vi "SaveOverlap.vi"(0 "ROI Cluster":T1, 1 "Intensity":dbl[][](array[numeric]), 2 "Auto Scale?":bool, 3 "Threshold (max)":dbl, 4 "Threshold (min)":dbl, 5 "G Data":dbl[][](array[numeric]), 6 "S Data":dbl[][](array[numeric]), 7 "error in":errorcluster, 8 "File Name":string, 9 "Index Name":string, 10 "Experiment Name":string, 11 "Time Stamp?":bool, 12 "Identify Name":string, 13 "Enable?":bool, 14 "path":path, 15 "Crop Pixels":u16=40) -> (20 "cancelled":bool, 27 "error out":errorcluster)   [LabVIEW 2018]
uses:
  <vilib>/picture/picture.llb/Draw True-Color Pixmap.vi
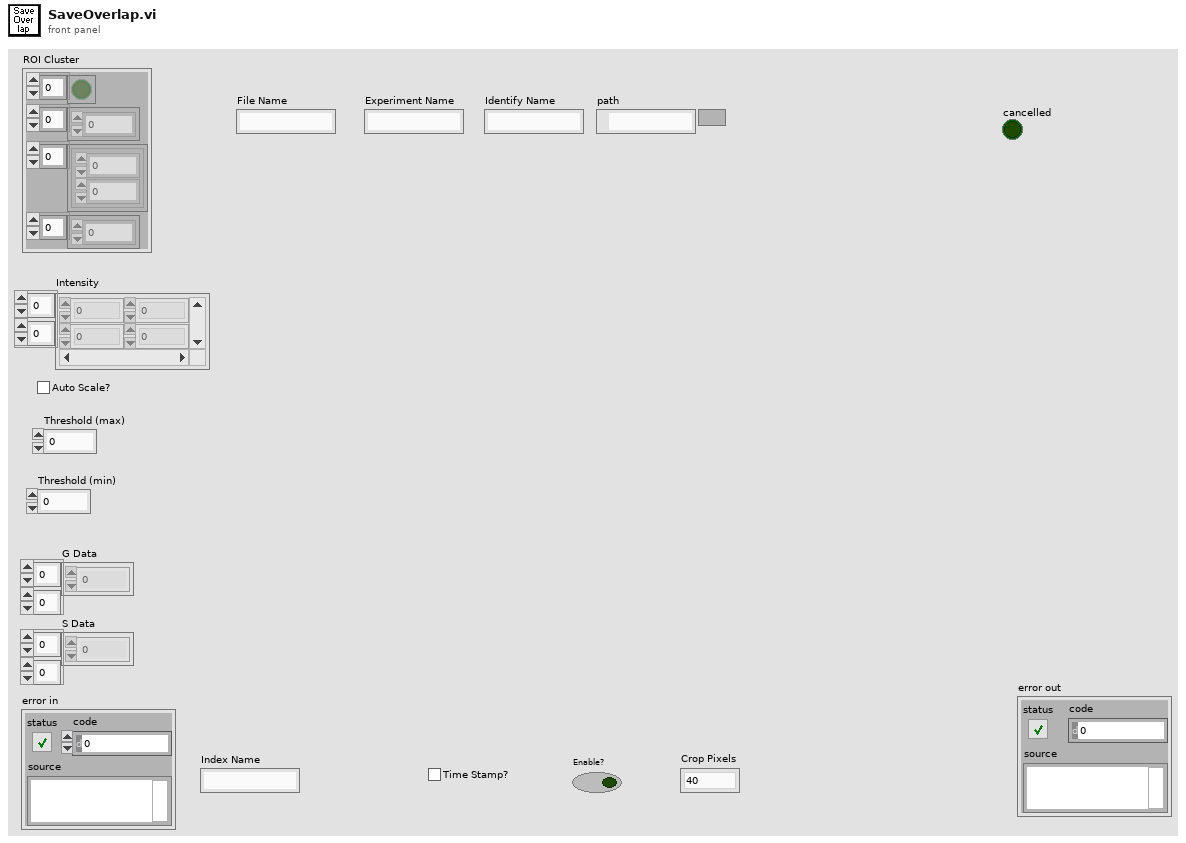
[diagram p1: front panel]
types:
  T1 = cluster{bool[], dbl[], cluster{dbl, dbl}[], u32[]}
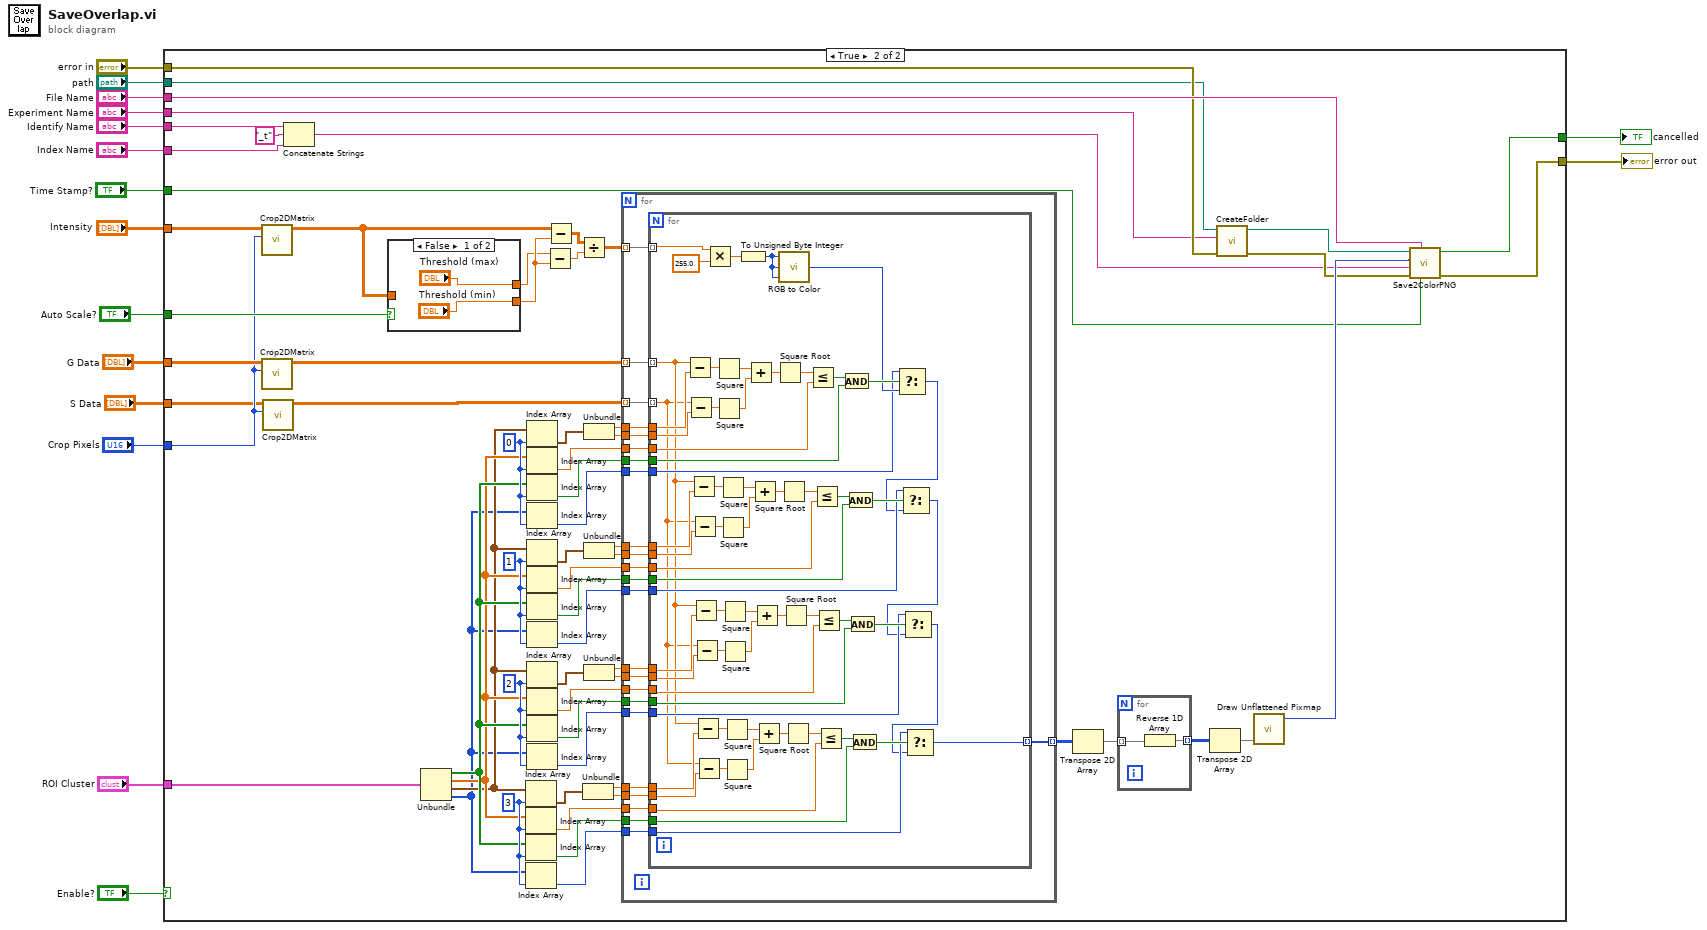
[diagram p0: block diagram]
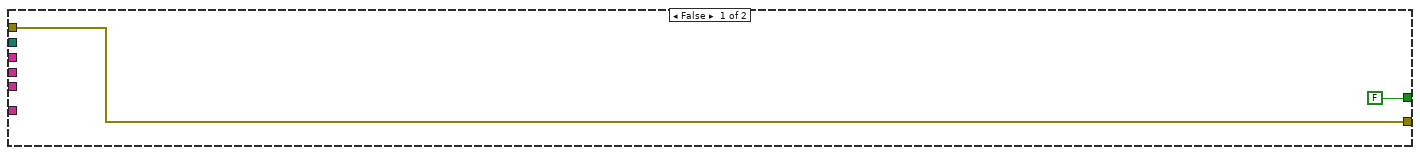
[diagram p2: hidden frame]
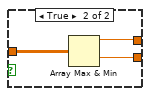
[diagram p3: hidden frame]
diagram:
  n1 = case shown="True" "Enable?" {
    tunnel: "S Data" -> [_ w30]
    tunnel: "G Data" -> [_ w33]
    tunnel: "Auto Scale?" -> [_ w78]
    tunnel: "Intensity" -> [_ w35]
    tunnel: "ROI Cluster" -> [_ w44]
    tunnel: "error in" -> [w17 w28]
    tunnel: [FALSE ("save cancelled") w38] -> w10
    tunnel: [w17 w39] -> w9
    tunnel: "path" -> [_ w27]
    tunnel: "File Name" -> [_ w37]
    tunnel: "Experiment Name" -> [_ w26]
    tunnel: "Identify Name" -> [_ w21]
    tunnel: "Time Stamp?" -> [_ w25]
    tunnel: "Crop Pixels" -> [_ w31]
    tunnel: "Index Name" -> [_ w20]
    frame False {
    }
    frame True {
      w47 = 3 ("index")
      w56 = 2 ("index")
      w61 = 1 ("index")
      w70 = 0 ("index")
      n2 = call "Crop2DMatrix.vi"("Crop Pixels"=w31, "Data"=w35) -> ("Cropped Data"=w34:dbl[][])  [unwired: 9 in]
      n3 = call "Crop2DMatrix.vi"("Crop Pixels"=w31, "Data"=w33) -> ("Cropped Data"=w32:dbl[][])  [unwired: 9 in]
      n4 = call "Crop2DMatrix.vi"("Crop Pixels"=w31, "Data"=w30) -> ("Cropped Data"=w29:dbl[][])  [unwired: 9 in]
      n5 = Concatenate Strings(w21, "_t" ("string"), w20) -> (w19:string)
      n6 = case shown="False" w78 {
        tunnel: w34 -> [_ w89]
        tunnel: ["Threshold (max)" w88] -> w76
        tunnel: ["Threshold (min)" w87] -> w77
        frame False {
        }
        frame True {
          n7 = Array Max & Min(array=w89) -> (max value=w88:dbl, min value=w87:dbl)  [unwired: 2 out]
        }
      }
      n8 = Unbundle(w44) -> (w43:bool[], w42:dbl[], w41:cluster{dbl, dbl}[], w40:u32[])
      n9 = Index Array(array=w41, index=w47) -> (element=w48:cluster{dbl, dbl})
      n10 = Index Array(array=w42, index=w47) -> (element=w49:dbl)
      n11 = Index Array(array=w43, index=w47) -> (element=w50:bool)
      n12 = Index Array(array=w40, index=w47) -> (element=w51:u32)
      n13 = Index Array(array=w41, index=w70) -> (element=w69:cluster{dbl, dbl})
      n14 = Index Array(array=w42, index=w70) -> (element=w68:dbl)
      n15 = Index Array(array=w43, index=w70) -> (element=w67:bool)
      n16 = Index Array(array=w40, index=w70) -> (element=w66:u32)
      n17 = Index Array(array=w41, index=w61) -> (element=w62:cluster{dbl, dbl})
      n18 = Index Array(array=w42, index=w61) -> (element=w63:dbl)
      n19 = Index Array(array=w43, index=w61) -> (element=w64:bool)
      n20 = Index Array(array=w40, index=w61) -> (element=w65:u32)
      n21 = Index Array(array=w41, index=w56) -> (element=w55:cluster{dbl, dbl})
      n22 = Index Array(array=w42, index=w56) -> (element=w54:dbl)
      n23 = Index Array(array=w43, index=w56) -> (element=w53:bool)
      n24 = Index Array(array=w40, index=w56) -> (element=w52:u32)
      n25 = Subtract(x=w76, y=w77) -> (x-y=w80:dbl)
      n26 = Subtract(x=w34, y=w77) -> (x-y=w79:dbl[][])
      n27 = Divide(x=w79, y=w80) -> (x/y=w72:dbl[][])
      n28 = Unbundle(w48) -> (w45:dbl, w46:dbl)
      n29 = Unbundle(w69) -> (w82:dbl, w81:dbl)
      n30 = Unbundle(w62) -> (w59:dbl, w60:dbl)
      n31 = Unbundle(w55) -> (w58:dbl, w57:dbl)
      n32 = for {
        tunnel: w32 -> [w113] mode=indexing
        tunnel: w29 -> [w112] mode=indexing
        tunnel: w82 -> [w111]
        tunnel: w81 -> [w110]
        tunnel: w68 -> [w109]
        tunnel: w72 -> [w108] mode=indexing
        tunnel: [w107] -> w71 mode=indexing
        tunnel: w67 -> [w106]
        tunnel: w66 -> [w105]
        tunnel: w59 -> [w100]
        tunnel: w60 -> [w101]
        tunnel: w63 -> [w102]
        tunnel: w64 -> [w103]
        tunnel: w65 -> [w104]
        tunnel: w58 -> [w99]
        tunnel: w57 -> [w98]
        tunnel: w54 -> [w97]
        tunnel: w53 -> [w96]
        tunnel: w52 -> [w95]
        tunnel: w45 -> [w90]
        tunnel: w46 -> [w91]
        tunnel: w49 -> [w92]
        tunnel: w50 -> [w93]
        tunnel: w51 -> [w94]
        n33 = for {
          tunnel: w113 -> [w119] mode=indexing
          tunnel: w112 -> [w118] mode=indexing
          tunnel: w111 -> [w176]
          tunnel: w110 -> [w175]
          tunnel: w109 -> [w174]
          tunnel: w108 -> [w164] mode=indexing
          tunnel: [w114] -> w107 mode=indexing
          tunnel: w106 -> [w162]
          tunnel: w105 -> [w159]
          tunnel: w100 -> [w150]
          tunnel: w101 -> [w149]
          tunnel: w102 -> [w148]
          tunnel: w103 -> [w147]
          tunnel: w104 -> [w146]
          tunnel: w99 -> [w129]
          tunnel: w98 -> [w128]
          tunnel: w97 -> [w127]
          tunnel: w96 -> [w126]
          tunnel: w95 -> [w125]
          tunnel: w90 -> [w124]
          tunnel: w91 -> [w123]
          tunnel: w92 -> [w122]
          tunnel: w93 -> [w121]
          tunnel: w94 -> [w120]
          # "Pixel Level"
          n34 = Subtract(x=w119, y=w176) -> (x-y=w173:dbl)
          n35 = Subtract(x=w118, y=w175) -> (x-y=w172:dbl)
          n36 = Subtract(x=w119, y=w150) -> (x-y=w151:dbl)
          n37 = Subtract(x=w118, y=w149) -> (x-y=w152:dbl)
          n38 = Subtract(x=w119, y=w129) -> (x-y=w145:dbl)
          n39 = Subtract(x=w118, y=w128) -> (x-y=w144:dbl)
          n40 = Subtract(x=w119, y=w124) -> (x-y=w130:dbl)
          n41 = Subtract(x=w118, y=w123) -> (x-y=w131:dbl)
          n42 = Multiply(x=w164, y=255.0) -> (x*y=w166:dbl)
          n43 = Square(x=w173) -> (x^2=w171:dbl)
          n44 = Square(x=w172) -> (x^2=w170:dbl)
          n45 = Square(x=w151) -> (x^2=w153:dbl)
          n46 = Square(x=w152) -> (x^2=w154:dbl)
          n47 = Square(x=w145) -> (x^2=w143:dbl)
          n48 = Square(x=w144) -> (x^2=w142:dbl)
          n49 = Square(x=w130) -> (x^2=w132:dbl)
          n50 = Square(x=w131) -> (x^2=w133:dbl)
          n51 = To Unsigned Byte Integer(number=w166) -> (unsigned 8bit integer=w167:u8)
          n52 = Add(x=w171, y=w170) -> (x+y=w169:dbl)
          n53 = Add(x=w153, y=w154) -> (x+y=w155:dbl)
          n54 = Add(x=w143, y=w142) -> (x+y=w141:dbl)
          n55 = Add(x=w132, y=w133) -> (x+y=w134:dbl)
          n56 = Square Root(x=w169) -> (sqrt(x)=w168:dbl)
          n57 = call <vilib>:"RGB to Color.vi"("B"=w167, "G"=w167, "R"=w167) -> ("Color"=w160:u32)
          n58 = Square Root(x=w155) -> (sqrt(x)=w156:dbl)
          n59 = Square Root(x=w141) -> (sqrt(x)=w140:dbl)
          n60 = Square Root(x=w134) -> (sqrt(x)=w135:dbl)
          n61 = Less Or Equal?(x=w168, y=w174) -> (x <= y?=w163:bool)
          n62 = Less Or Equal?(x=w156, y=w148) -> (x <= y?=w157:bool)
          n63 = Less Or Equal?(x=w140, y=w127) -> (x <= y?=w139:bool)
          n64 = Less Or Equal?(x=w135, y=w122) -> (x <= y?=w136:bool)
          n65 = And(x=w163, y=w162) -> (x .and. y?=w161:bool)
          n66 = And(x=w157, y=w147) -> (x .and. y?=w158:bool)
          n67 = And(x=w139, y=w126) -> (x .and. y?=w138:bool)
          n68 = And(x=w136, y=w121) -> (x .and. y?=w137:bool)
          n69 = Select(t=w159, s=w161, f=w160) -> (s? t:f=w117:u32)
          n70 = Select(t=w146, s=w158, f=w117) -> (s? t:f=w116:u32)
          n71 = Select(t=w125, s=w138, f=w116) -> (s? t:f=w115:u32)
          n72 = Select(t=w120, s=w137, f=w115) -> (s? t:f=w114:u32)
        }
      }
      n73 = Transpose 2D Array(2D array=w71) -> (transposed array=w75:u32[][])
      n74 = for {
        tunnel: w75 -> [w84] mode=indexing
        tunnel: [w83] -> w74 mode=indexing
        n75 = Reverse 1D Array(array=w84) -> (reversed array=w83:u32[])
      }
      n76 = Transpose 2D Array(2D array=w74) -> (transposed array=w73:u32[][])
      n77 = call "CreateFolder.vi"("error in (no error)"=w28, "name"=w26, "base path"=w27) -> ("error out"=w23:errorcluster, "path out"=w24:path)  [unwired: 7 in]
      n78 = call-poly <vilib>:"Draw Unflattened Pixmap.vi"("data (RGB format)"=w73) -> ("new picture"=w36:picture)  [unwired: 8 in]
      n79 = call "Save2ColorPNG.vi"("Time Stamp?"=w25, "File Name Prefix"=w37, "error in"=w23, "Identify Name"=w19, "Data Picture"=w36, "Parent Directory"=w24) -> ("error out"=w39:errorcluster, "cancelled"=w38:bool)  [unwired: 4 in]
    }
  }
  "cancelled" <- w10
  "error out" <- w9
